vi "Display_EEPROM.vi"() -> ()   [LabVIEW 2019]
uses:
  D2XX_Functions/D2XX_Functions.lvlib
panel:
  out "output cluster":T1
  out "error out":errorcluster
  in  "error in (no error)":errorcluster
  out "FT_Status":u32(ring) items=["FT_OK", "FT_INVALID_HANDLE", "FT_DEVICE_NOT_FOUND", "FT_DEVICE_NOT_OPENED", "FT_IO_ERROR", "FT_INSUFFICIENT_RESOURCES", "FT_INVALID_PARAMETER", "FT_INVALID_BAUD_RATE", "FT_DEVICE_NOT_OPENED_FOR_ERASE", "FT_DEVICE_NOT_OPENED_FOR_WRITE", "FT_FAILED_TO_WRITE_DEVICE", "FT_EEPROM_READ_FAILED", "FT_EEPROM_WRITE_FAILED", "FT_EEPROM_ERASE_FAILED", "FT_EEPROM_NOT_PRESENT", "FT_EEPROM_NOT_PROGRAMMED", "FT_INVALID_ARGS", "FT_NOT_SUPPORTED", "FT_OTHER_ERROR"]
  out "Port Index":string
  out "Device Description":string
  out "FT_Status 2":u32(ring) items=["FT_OK", "FT_INVALID_HANDLE", "FT_DEVICE_NOT_FOUND", "FT_DEVICE_NOT_OPENED", "FT_IO_ERROR", "FT_INSUFFICIENT_RESOURCES", "FT_INVALID_PARAMETER", "FT_INVALID_BAUD_RATE", "FT_DEVICE_NOT_OPENED_FOR_ERASE", "FT_DEVICE_NOT_OPENED_FOR_WRITE", "FT_FAILED_TO_WRITE_DEVICE", "FT_EEPROM_READ_FAILED", "FT_EEPROM_WRITE_FAILED", "FT_EEPROM_ERASE_FAILED", "FT_EEPROM_NOT_PRESENT", "FT_EEPROM_NOT_PROGRAMMED", "FT_INVALID_ARGS", "FT_NOT_SUPPORTED", "FT_OTHER_ERROR"]
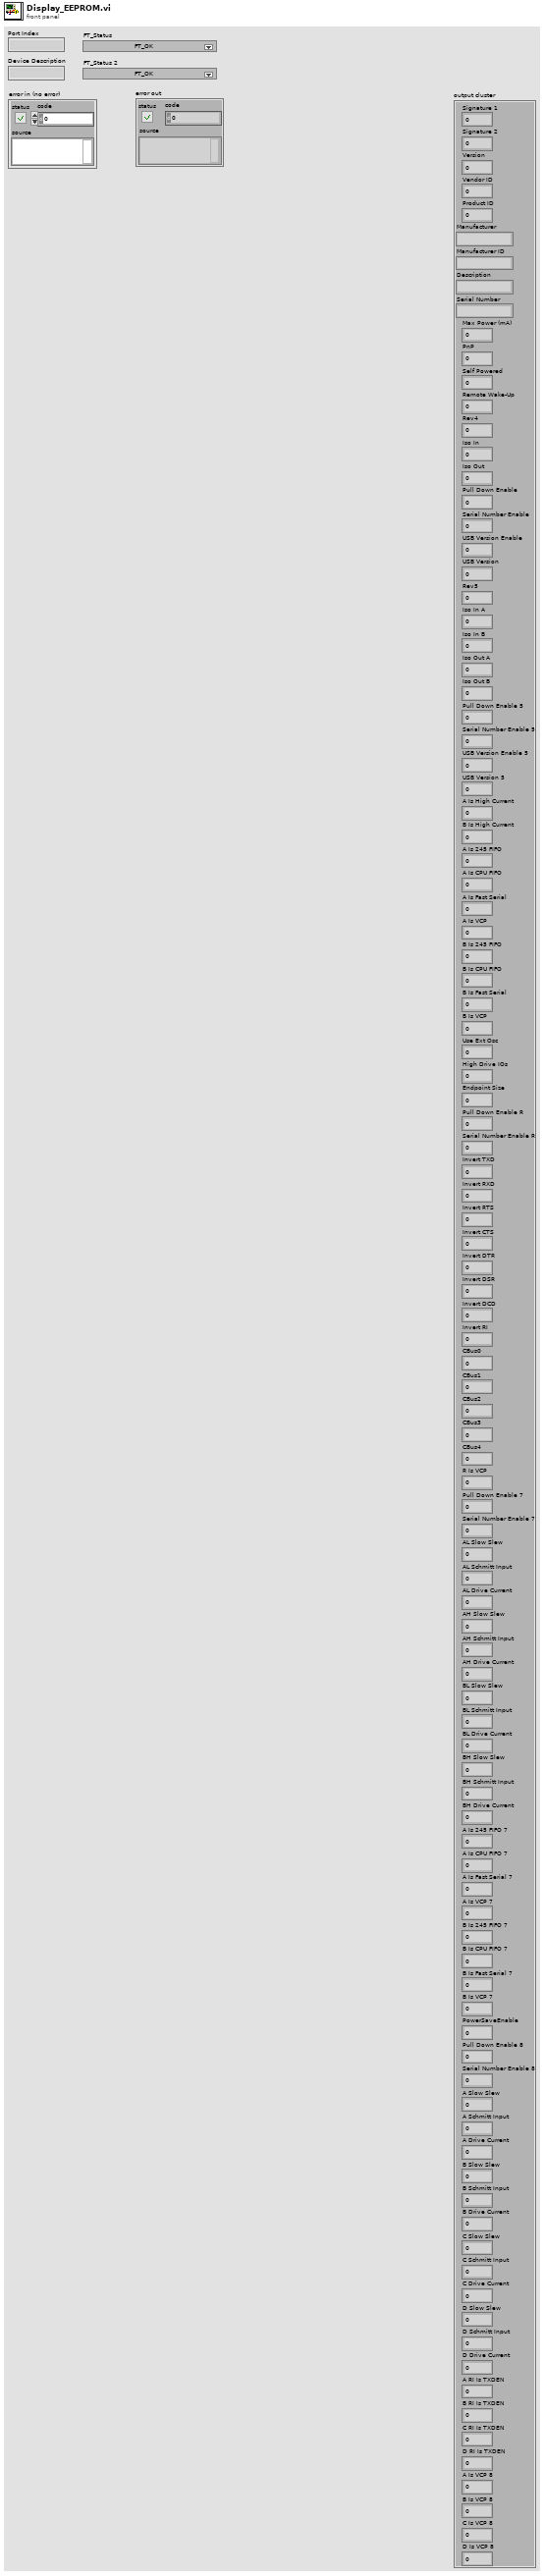
[diagram p1: front panel]
types:
  T1 = cluster{"Signature 1":u32, "Signature 2":u32, "Version":u32, "Vendor ID":u16, "Product ID":u16, "Manufacturer":string, "Manufacturer ID":string, "Description":string, "Serial Number":string, "Max Power (mA)":u16, "PnP":u16, "Self Powered":u16, "Remote Wake-Up":u16, "Rev4":u8, "Iso In":u8, "Iso Out":u8, "Pull Down Enable":u8, "Serial Number Enable":u8, "USB Version Enable":u8, "USB Version":u16, "Rev5":u8, "Iso In A":u8, "Iso In B":u8, "Iso Out A":u8, "Iso Out B":u8, "Pull Down Enable 5":u8, "Serial Number Enable 5":u8, "USB Version Enable 5":u8, "USB Version 5":u16, "A Is High Current":u8, "B Is High Current":u8, "A Is 245 FIFO":u8, "A Is CPU FIFO":u8, "A Is Fast Serial":u8, "A Is VCP":u8, "B Is 245 FIFO":u8, "B Is CPU FIFO":u8, "B Is Fast Serial":u8, "B Is VCP":u8, "Use Ext Osc":u8, "High Drive IOs":u8, "Endpoint Size":u8, "Pull Down Enable R":u8, "Serial Number Enable R":u8, "Invert TXD":u8, "Invert RXD":u8, "Invert RTS":u8, "Invert CTS":u8, "Invert DTR":u8, "Invert DSR":u8, "Invert DCD":u8, "Invert RI":u8, "CBus0":u8, "CBus1":u8, "CBus2":u8, "CBus3":u8, "CBus4":u8, "R Is VCP":u8, "Pull Down Enable 7":u8, "Serial Number Enable 7":u8, "AL Slow Slew":u8, "AL Schmitt Input":u8, "AL Drive Current":u8, "AH Slow Slew":u8, "AH Schmitt Input":u8, "AH Drive Current":u8, "BL Slow Slew":u8, "BL Schmitt Input":u8, "BL Drive Current":u8, "BH Slow Slew":u8, "BH Schmitt Input":u8, "BH Drive Current":u8, "A Is 245 FIFO 7":u8, "A Is CPU FIFO 7":u8, "A Is Fast Serial 7":u8, "A Is VCP 7":u8, "B Is 245 FIFO 7":u8, "B Is CPU FIFO 7":u8, "B Is Fast Serial 7":u8, "B Is VCP 7":u8, "PowerSaveEnable":u8, "Pull Down Enable 8":u8, "Serial Number Enable 8":u8, "A Slow Slew":u8, "A Schmitt Input":u8, "A Drive Current":u8, "B Slow Slew":u8, "B Schmitt Input":u8, "B Drive Current":u8, "C Slow Slew":u8, "C Schmitt Input":u8, "C Drive Current":u8, "D Slow Slew":u8, "D Schmitt Input":u8, "D Drive Current":u8, "A RI Is TXDEN":u8, "B RI Is TXDEN":u8, "C RI Is TXDEN":u8, "D RI Is TXDEN":u8, "A Is VCP 8":u8, "B Is VCP 8":u8, "C Is VCP 8":u8, "D Is VCP 8":u8}
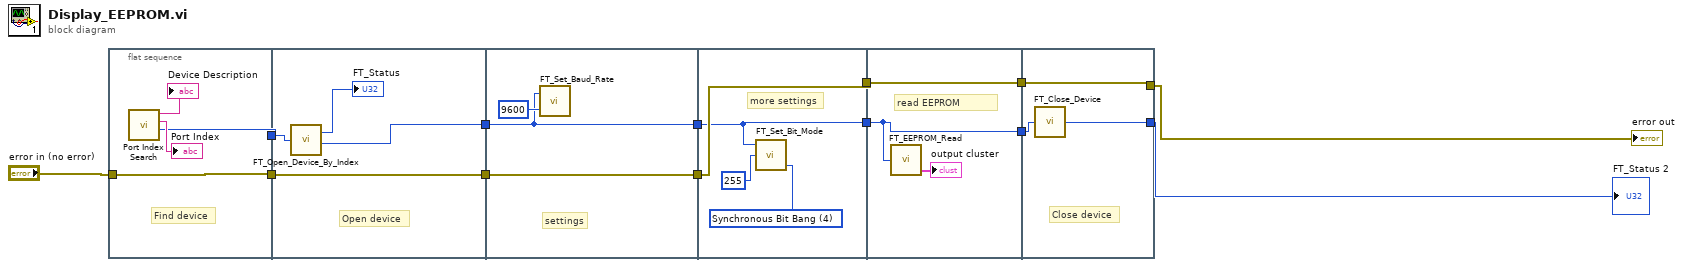
[diagram p0: block diagram]
diagram:
  n1 = flat-sequence {
    tunnel: [w14] -> w13
    tunnel: "error in (no error)" -> [w15]
    tunnel: [w15] -> w12
    tunnel: w13 -> [w20]
    tunnel: [w18] -> w11
    tunnel: [w19] -> w10
    tunnel: w12 -> [w19]
    tunnel: [w22] -> w9
    tunnel: w11 -> [w22]
    tunnel: [w23] -> w8
    tunnel: w10 -> [w23]
    tunnel: w9 -> [w25]
    tunnel: w8 -> [w26]
    tunnel: [w26] -> w4
    tunnel: [w25] -> w3
    tunnel: w4 -> [w31]
    tunnel: [w31] -> w2
    tunnel: w3 -> [w30]
    tunnel: [w30] -> w1
    tunnel: [w34] -> w7
    tunnel: [w33] -> w5
    tunnel: w2 -> [w33]
    tunnel: w1 -> [w32]
    frame #0 {
      # "Find device"
      n2 = call "Port Index Search.vi"() -> ("Decimal Port Index"=w14:i32, "Port Index"=→"Port Index":string, "Device Description"=→"Device Description":string)  [unwired: 8 in, 1 out]
    }
    frame #1 {
      # "Open device"
      n3 = call "FT_Open_Device_By_Index.vi"("Device Index"=w20) -> ("FT_Status"=→"FT_Status":u32, "Handle"=w18:u32)
    }
    frame #2 {
      # "settings"
      n4 = call "FT_Set_Baud_Rate.vi"("Baud Rate"=u32 9600, "Handle"=w22) -> ()  [unwired: 1 out]
    }
    frame #3 {
      w28 = u8 4 items=["Reset Bit Mode"=0, "Asynchronous Bit Bang"=1, "MPSSE"=2, "Synchronous Bit Bang"=4, "MCU Host Bus Emulation"=8, "Fast Opto-Isolated Serial"=16, "CBUS Bit Bang"=32, "Single Channel 245 Synchronous FIFO"=64] ("Bit Mode")
      # "more settings"
      n5 = call "FT_Set_Bit_Mode.vi"("Bit Mode"=w28, "Bit Mode Mask"=u8 255, "Handle"=w25) -> ()  [unwired: 1 out]
    }
    frame #4 {
      # "read EEPROM"
      n6 = call "FT_EEPROM_Read.vi"("Handle"=w30) -> ("output cluster"=→"output cluster":T1)  [unwired: 2 out]
    }
    frame #5 {
      # "Close device"
      n7 = call "FT_Close_Device.vi"("Handle"=w32) -> ("FT_Status"=w34:u32)
    }
  }
  "FT_Status 2" <- w7
  "error out" <- w5
